vi "Generate Test Sequence.vi"(10 "Number of Iterations":i32) -> (2 "Test Sequence":T1[][](array[typedef]))   [LabVIEW 2017]
uses:
  Working Demo Phase/states.ctl
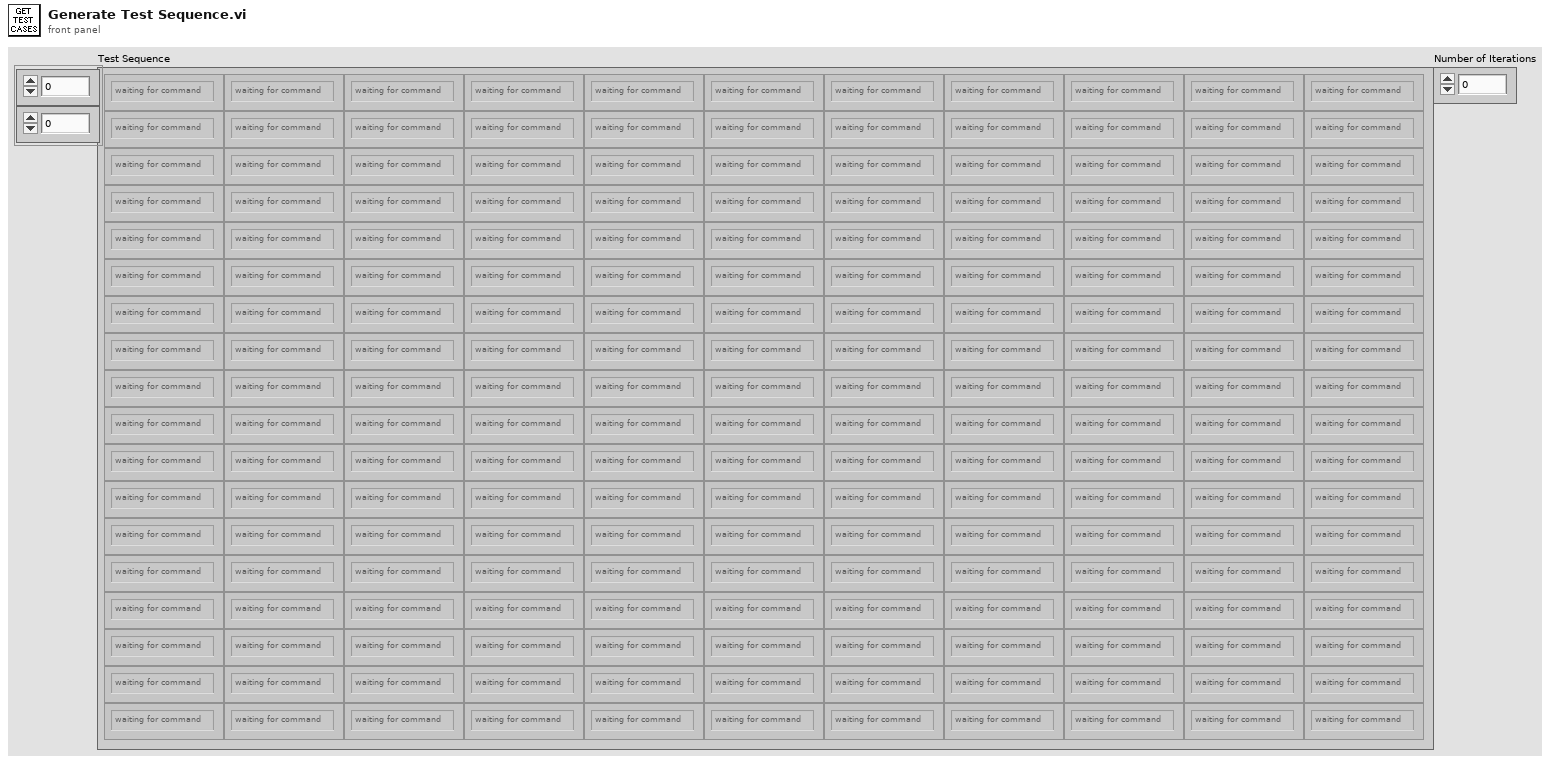
[diagram p1: front panel]
types:
  T1 = typedef "states.ctl" = enum16{"waiting for command", "go to ground floor", "go to floor 1", "go to floor 2", "drop cart"}
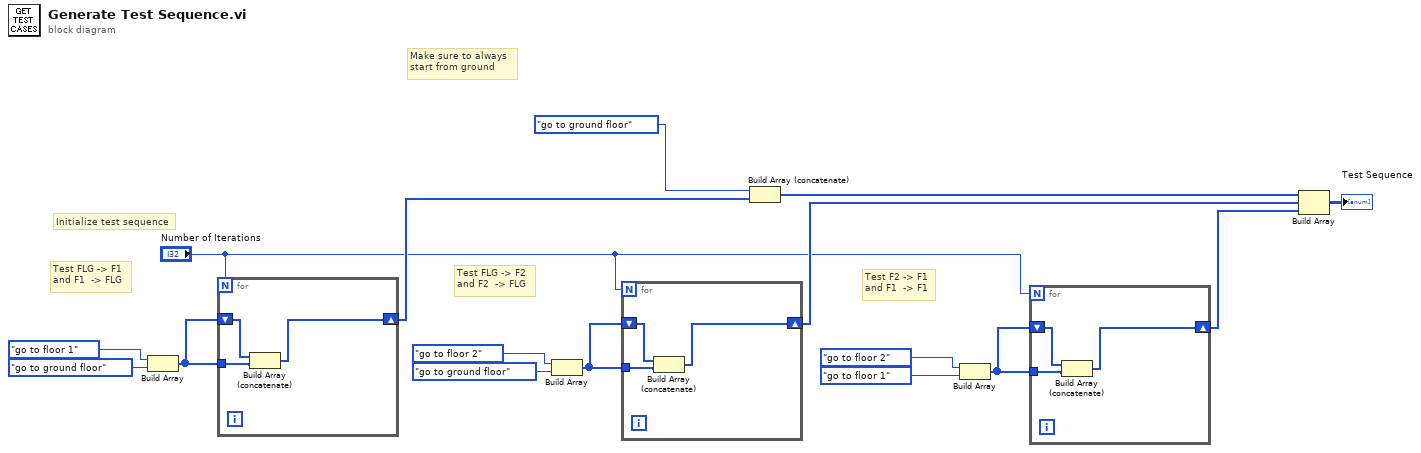
[diagram p0: block diagram]
diagram:
  # "Make sure to always\nstart from ground"
  # "Test F2 -> F1\nand F1  -> F1"
  # "Test FLG -> F2\nand F2  -> FLG"
  # "Test FLG -> F1\nand F1  -> FLG"
  # "Initialize test sequence"
  n1 = Build Array(states."go to floor 1", states."go to ground floor") -> (w16:T1[])
  n2 = for {
    N: "Number of Iterations" -> [_]
    shift-right: [w17] -> w7
    shift-left: w16 -> [w19]
    tunnel: w16 -> [w18]
    n3 = Build Array (concatenate)(w19, w18) -> (w17:T1[])
  }
  n4 = Build Array(states."go to floor 2", states."go to ground floor") -> (w13:T1[])
  n5 = for {
    N: "Number of Iterations" -> [_]
    shift-right: [w20] -> w6
    shift-left: w13 -> [w22]
    tunnel: w13 -> [w21]
    n6 = Build Array (concatenate)(w22, w21) -> (w20:T1[])
  }
  n7 = Build Array (concatenate)(states."go to ground floor", w7) -> (w2:T1[])
  n8 = Build Array(states."go to floor 2", states."go to floor 1") -> (w10:T1[])
  n9 = for {
    N: "Number of Iterations" -> [_]
    shift-right: [w23] -> w5
    shift-left: w10 -> [w25]
    tunnel: w10 -> [w24]
    n10 = Build Array (concatenate)(w25, w24) -> (w23:T1[])
  }
  n11 = Build Array(w2, w6, w5) -> (→"Test Sequence":T1[][])
